vi "DirectoriesToIgnore.vi"() -> (2 "IgnoredDirectories[]":string[](array[string])=["C:\\\\Program Files\\\\"])   [LabVIEW 2021, in "Converter Reusables.lvlib"]
uses:
  Converter Reusables.lvlib
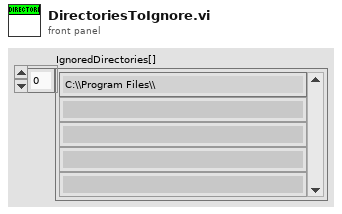
[diagram p1: front panel]
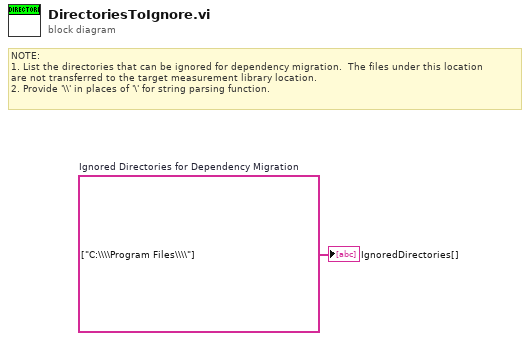
[diagram p0: block diagram]
diagram:
  w1 = string[] ["C:\\\\Program Files\\\\"]  # Ignored Directories for Dependency Migration
  # "NOTE:\n1. List the directories that can be ignored for dependency migration.  The files under this location\nare not transferred to the target measurement library location.\n2. Provide '\\\\' in places of '\\' for string parsing function."
  "IgnoredDirectories[]" <- w1
